vi "CreateSelfReference.vi"(8 "error in (no error)":errorcluster, 11 "SignalSenderLoop":refnum<class "SignalSenderLoop.lvclass">) -> (0 "error out":errorcluster, 3 "SignalSenderLoop out":refnum<class "SignalSenderLoop.lvclass">)   [LabVIEW 2020, in "ECU_Diagnose.lvlib" / "SignalSenderLoop.lvclass"]
doc: "JKI State Machine Objects (SMO) 1.0.0.5\nJKI - JKI\nCopyright (c) 2016, JKI"
uses:
  SignalSenderLoop.lvclass
  SignalSenderLoop.lvclass/SignalSenderLoop.ctl
  <vilib>/JKI/JKI SMO/SMO/SMO.lvclass
panel:
  # "For instructions on how to use the JKI State Machine Objects, examples and video tutorials, visit:\nhttp://jki.net/state-machine-objects/\n\nJKI State Machine Objects™\nhttp://jki.net/state-machine-objects/\nCopyright (C) 2005-2015, JKI <info@jki.net>\nALL RIGHTS RESERVED"
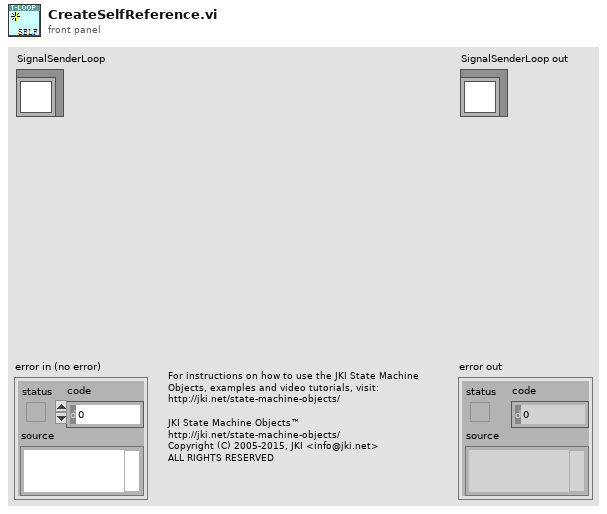
[diagram p1: front panel]
types:
  T1 = typedef "ECU_Diagnose.lvlib/SignalSenderLoop.lvclass/PrivateData--Ref.ctl" = refnum<data-value>
  T2 = typedef "ECU_Diagnose.lvlib/SignalSenderLoop.lvclass/PrivateData--Cluster.ctl" = cluster{"Public Events":T3, "Setpoint":T4, "Private Events":T5, "SignalFrameSet":T6}
  T3 = typedef "ECU_Diagnose.lvlib/SignalSenderLoop.lvclass/PublicEvents--Cluster.ctl" = cluster{"Setpoint Changed":refnum<user-event>, "Value Changed":refnum<user-event>}
  T4 = typedef "ECU_Diagnose.lvlib/SignalSenderLoop.lvclass/Data.ctl" = dbl
  T5 = typedef "ECU_Diagnose.lvlib/SignalSenderLoop.lvclass/PrivateEvents--Cluster.ctl" = cluster{"AsyncMethod":refnum<user-event>, "SignalCMDArry":refnum<user-event>}
  T6 = typedef "ECU_Diagnose.lvlib/SignalSenderLoop.lvclass/SignalFrameSet.ctl" = cluster{"Port_No.":refnum<k21>, "计数Count":bool, "校验CheckSum":bool, "MessageFrame":refnum<k21>, "校验算法名称":string}
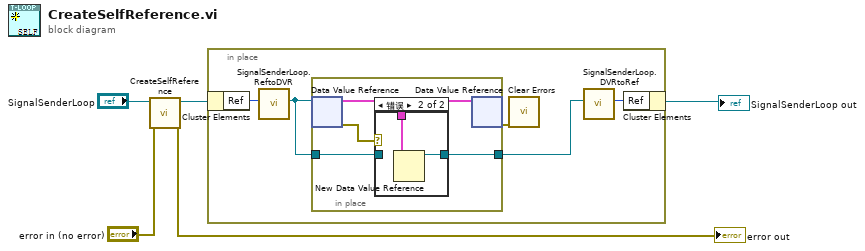
[diagram p0: block diagram]
diagram:
  n1 = call-parent "CreateSelfReference.vi"("error in (no error)"="error in (no error)", "SMO"="SignalSenderLoop") -> ("error out"=→"error out":errorcluster, "SMO out"=w4:refnum<class "SignalSenderLoop.lvclass">)  [unwired: 8 in]
  n2 = in-place {
    n3 = in-place-cluster #1(w4) -> ("Ref"=w10:u32)
    n4 = call "SignalSenderLoop.ReftoDVR.vi"("Ref"=w10) -> ("Ref"=w9:T1)  [unwired: 10 in]
    n5 = in-place {
      in-place-border: [w14] -> w7
      in-place-border: w9 -> [w11]
      n6 = in-place-dvr #2(w9) -> (w13:T2, w12:errorcluster)
      n7 = case shown="错误" w12 {
        tunnel: [w15 w17] -> w14
        tunnel: w13 -> [_ w16]
        tunnel: w11 -> [w15 _]
        frame No Error {
        }
        frame Error {
          n8 = New Data Value Reference(data value=w16) -> (data value reference=w17:refnum<data-value>)  [unwired: 1 in, 1 out]
        }
      }
      n9 = in-place-dvr #2(w13) -> (w6:errorcluster)  [unwired: 1 out]
    }
    n10 = call <vilib>:"Clear Errors.vi"("error in (no error)"=w6) -> ()  [unwired: 5 in, 2 out]
    n11 = call "SignalSenderLoop.DVRtoRef.vi"("Ref"=w7) -> ("Ref"=w8:u32)  [unwired: 10 in]
    n12 = in-place-cluster #1("Ref"=w8) -> (→"SignalSenderLoop out":refnum<class "SignalSenderLoop.lvclass">)
  }
